vi "sensor config set v2.vi"(9 "value":u32, 10 "setting":u32(ring) items=["CONFIG_V2_OUTPUT_RATE", "CONFIG_V2_OUTPUT_RATE_WIRELESS_DIVIDER", "CONFIG_V2_ENABLE_ACCEL", "CONFIG_V2_ENABLE_GYRO", "CONFIG_V2_ENABLE_MAG", "CONFIG_V2_ENABLE_PRESSURE", "CONFIG_V2_FILE_FORMAT", "CONFIG_V2_ENABLE_SI_SD_DATA_LOGGING", "CONFIG_V2_ENABLE_RAW_SD_DATA_LOGGING", "CONFIG_V2_WIRELESS_PROTOCOL", "CONFIG_V2_WIRELESS_CHANNEL", "CONFIG_V2_WIRELESS_TX_POWER", "CONFIG_V2_WIRELESS_LATENCY_MS", "CONFIG_V2_WIRELESS_GROUP_CODE", "CONFIG_V2_WIRELESS_TX_MASK", "CONFIG_V2_WIRELESS_TARGET_AP_ID", "CONFIG_V2_WIRELESS_DEBUG_CONTROL", "CONFIG_V2_FILTER_MODE", "CONFIG_V2_FILTER_MAX_LATENCY_MS", "CONFIG_V2_SD_CARD_BUFFERING", "CONFIG_V2_BATTERY_CUTOFF", "CONFIG_V2_LED_MODE", "CONFIG_V2_BUTTON_MODE", "CONFIG_V2_EXTERNAL_COMMUNICATIONS_MODE", "CONFIG_V2_LCD_DISPLAY_ENABLE", "CONFIG_V2_LCD_DISPLAY_ANGLE", "CONFIG_V2_NUMBER_OF_APS", "CONFIG_V2_DEBUG_LCD_ENABLE", "CONFIG_V2_ENABLE_USB_CDC_ACM_VCOM", "CONFIG_V2_ENABLE_AP_DATA_STREAMING", "CONFIG_V2_UNUSED2", "CONFIG_V2_UNUSED3", "CONFIG_V2_UNUSED4", "CONFIG_V2_DISABLE_CALIBRATION_DATA", "CONFIG_V2_RAW_RATE_OVERRIDE_ACCEL_MID", "CONFIG_V2_RAW_RATE_OVERRIDE_ACCEL_HIGH", "CONFIG_V2_RAW_RATE_OVERRIDE_GYRO", "CONFIG_V2_RAW_RATE_OVERRIDE_MAG", "CONFIG_V2_RANGE_OVERRIDE_ACCEL_MID", "CONFIG_V2_RANGE_OVERRIDE_GYRO", "CONFIG_V2_RANGE_OVERRIDE_MAG", "CONFIG_V2_LOGGING_BEHAVIOR", "CONFIG_V2_ENABLE_RANGING", "CONFIG_V2_SENSOR_INDEX", "CONFIG_V2_SENSOR_COUNT", "CONFIG_V2_MOUNT_MODE", "CONFIG_V2_WIRELESS_MESH_CHANNEL", "CONFIG_V2_WIRELESS_DOCKING_BEHAVIOR", "CONFIG_V2_STANDBY_MODE", "CONFIG_V2_VALUE_LAST_ELEMENT"], 11 "h":u32) -> (2 "function return":i32, 3 "h out":u32)   [LabVIEW 2019, in "apdm.lvlib"]
doc: "APDM_EXPORT int apdm_sensor_config_set_v2(apdm_device_handle_t h, const config_value_t setting, const uint32_t value);"
uses:
  apdm.lvlib
  Lee Lab/CP FES Walking 2018/Code/Working/LabVIEW/apdm.dll
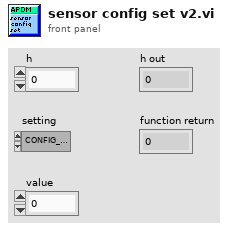
[diagram p1: front panel]
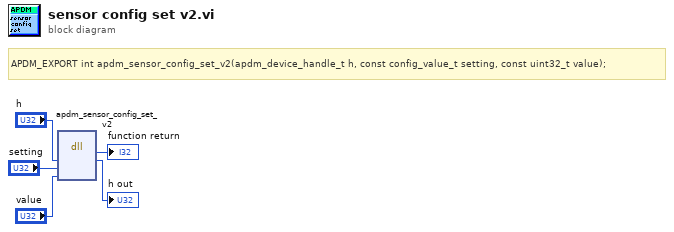
[diagram p0: block diagram]
diagram:
  # "APDM_EXPORT int apdm_sensor_config_set_v2(apdm_device_handle_t h, const config_value_t setting, const uint32_t value);"
  n1 = dll-call lib="C:/Users/jfalesi/Dropbox/Lee Lab/CP FES Walking 2018/Code/Working/LabVIEW/apdm.*" fn="apdm_sensor_config_set_v2"("h"="h", "setting"="setting", "value"="value") -> (→"function return":i32, "h"=→"h out":u32)  [unwired: 5 in, 2 out]
